vi "BRig_dataExp_T_Wrong.vi"() -> (2 "output_T_Wrong":i32)   [LabVIEW 2014]
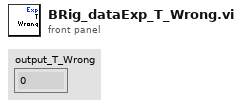
[diagram p1: front panel]
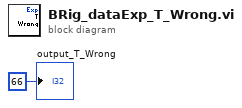
[diagram p0: block diagram]
diagram:
  "output_T_Wrong" <- 66 ("output_iBlock")
